vi "Timing Edit Transfer.vi"(9 "Application Timing and Logging Old":T1, 11 "Application Timing and Logging New":T1) -> (3 "Application Timing and Logging Out":T1)   [LabVIEW 2013]
uses:
  Application/Timing & Logging Parameters.ctl
  Application/Timing Parameters.ctl
panel:
  # "Interval is in Seconds\nRate is in Samples per Second"
  # "Interval is in Seconds\nRate is in Samples per Second"
  # "Interval is in Seconds\nRate is in Samples per Second"
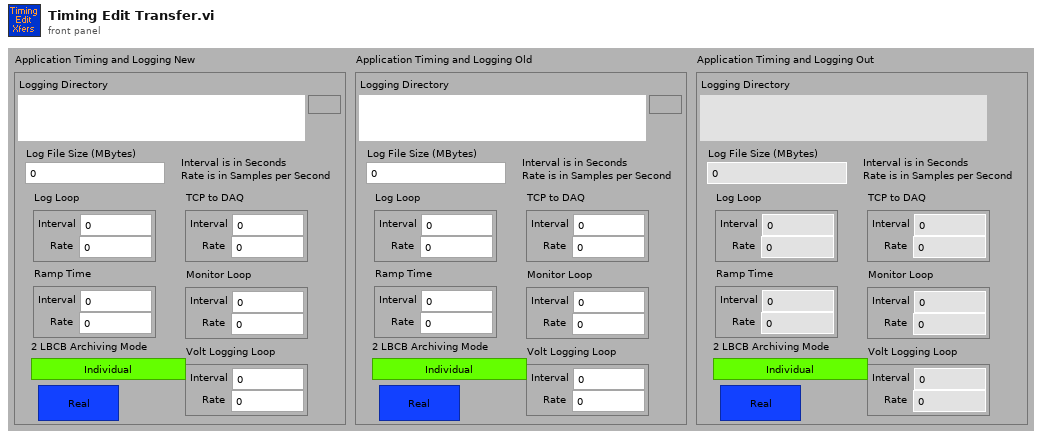
[diagram p1: front panel]
types:
  T1 = typedef "Timing & Logging Parameters.ctl" = cluster{"Monitor Loop":T2, "Ramp Time":T2, "Log Loop":T2, "TCP to DAQ":T2, "Logging Directory":path, "Log File Size (MBytes)":i64, "Volt Logging Loop":T2, "2 LBCB Archiving Mode":bool, "Fake":bool}
  T2 = typedef "Timing Parameters.ctl" = cluster{"Interval":dbl, "Rate ":dbl}
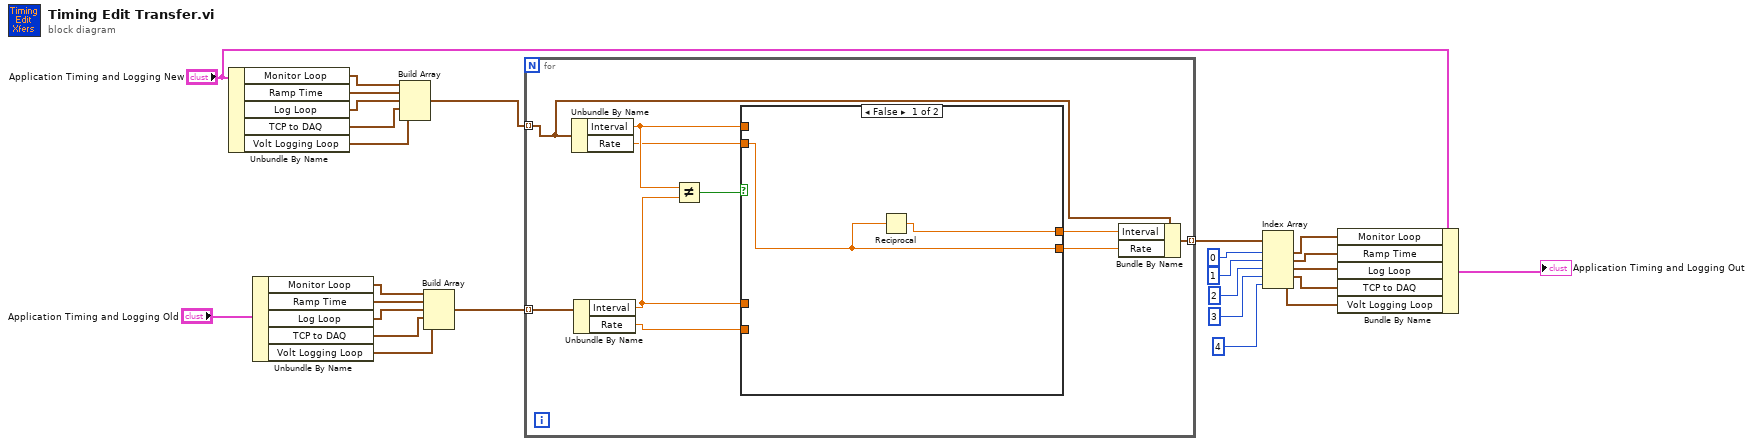
[diagram p0: block diagram]
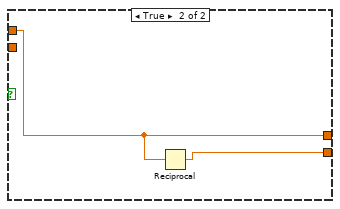
[diagram p2: hidden frame]
diagram:
  n1 = Unbundle By Name("Application Timing and Logging New") -> ("Monitor Loop"=w26:T2, "Ramp Time"=w25:T2, "Log Loop"=w24:T2, "TCP to DAQ"=w23:T2, "Volt Logging Loop"=w22:T2)
  n2 = Unbundle By Name("Application Timing and Logging Old") -> ("Monitor Loop"=w21:T2, "Ramp Time"=w20:T2, "Log Loop"=w19:T2, "TCP to DAQ"=w18:T2, "Volt Logging Loop"=w17:T2)
  n3 = Build Array(w26, w25, w24, w23, w22) -> (w15:T2[])
  n4 = Build Array(w21, w20, w19, w18, w17) -> (w14:T2[])
  n5 = for {
    tunnel: w15 -> [w34] mode=indexing
    tunnel: w14 -> [w36] mode=indexing
    tunnel: [w27] -> w13 mode=indexing
    n6 = Unbundle By Name(w34) -> ("Interval"=w33:dbl, "Rate"=w32:dbl)
    n7 = Unbundle By Name(w36) -> ("Interval"=w31:dbl, "Rate"=w30:dbl)
    n8 = Not Equal?(x=w33, y=w31) -> (x != y?=w35:bool)
    n9 = case shown="False" w35 {
      tunnel: w33 -> [_ w40]
      tunnel: w32 -> [w38 _]
      tunnel: w31 -> [_ _]
      tunnel: w30 -> [_ _]
      tunnel: [w37 w40] -> w29
      tunnel: [w38 w39] -> w28
      frame False {
        n10 = Reciprocal(x=w38) -> (1/x=w37:dbl)
      }
      frame True {
        n11 = Reciprocal(x=w40) -> (1/x=w39:dbl)
      }
    }
    n12 = Bundle By Name(cluster=w34, "Interval"=w29, "Rate"=w28) -> (w27:T2)
  }
  n13 = Index Array(array=w13, index #1=0 ("index"), index #2=1 ("index"), index #3=2 ("index"), index #4=3 ("index"), index #5=4 ("index")) -> (element #1=w7:T2, element #2=w6:T2, element #3=w5:T2, element #4=w4:T2, element #5=w2:T2)
  n14 = Bundle By Name(cluster="Application Timing and Logging New", "Monitor Loop"=w7, "Ramp Time"=w6, "Log Loop"=w5, "TCP to DAQ"=w4, "Volt Logging Loop"=w2) -> (→"Application Timing and Logging Out":T1)
